vi "Write Housekeeping TS.vi"(8 "error in (no error)":errorcluster, 10 "Housekeeping":i64, 11 "CIFCorePlugin in":refnum<class "CIFCorePlugin.lvclass">) -> (0 "error out":errorcluster, 3 "CIFCorePlugin out":refnum<class "CIFCorePlugin.lvclass">)   [LabVIEW 2021, in "CIFCorePlugin.lvclass"]
doc: "Update the timestamp. Time is U64, absolute time in nS in the appropriate clockID configured for the plugin. If a 0 is wired it will automatically get the current time."
uses:
  CIFCorePlugin.lvclass
  CIFCorePlugin.lvclass/CIFCorePlugin.ctl
  CIFUtilities/CIFClocks/Time Conversion/LabVIEW Time to UTC Time.vi
  Common/Utilities/Add Error.vi
  Common/Utilities/Append Error Location.vi
  <vilib>/CIF Foundation/CIF Utilities/Time/Time_CIF_U.lvlib
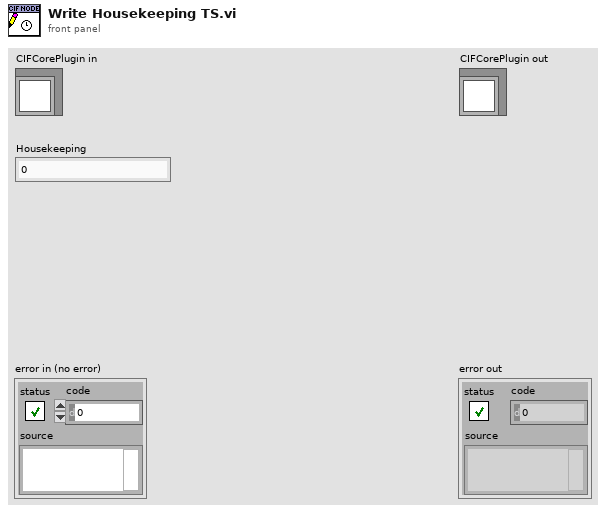
[diagram p1: front panel]
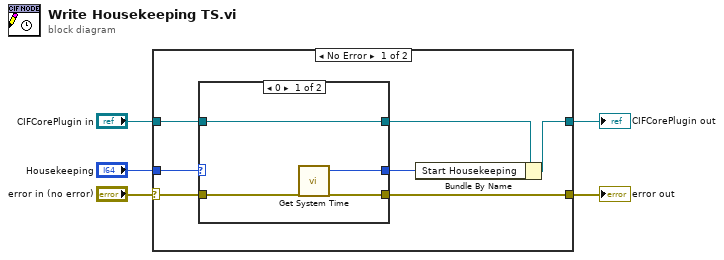
[diagram p0: block diagram]
diagram:
  n1 = case shown="No Error" "error in (no error)" {
    selector: "error in (no error)" -> [w10 w19]
    tunnel: [w6 w19] -> w4
    tunnel: [w12 w20] -> w2
    tunnel: "CIFCorePlugin in" -> [w9 w20]
    tunnel: "Housekeeping" -> [w11 _]
    frame No Error {
      n2 = case shown="0" w11 {
        selector: w11 -> [_ w17]
        tunnel: w10 -> [w13 w16]
        tunnel: w9 -> [w15 w18]
        tunnel: [w15 w18] -> w8
        tunnel: [w14 w17] -> w7
        tunnel: [w13 w16] -> w6
        frame 0 {
          n3 = call <vilib>:"Get System Time.vi"() -> ("Time (ns)"=w14:i64)  [unwired: 5 in]
        }
        frame 1, Default {
        }
      }
      n4 = Bundle By Name(cluster=w8, "Start Housekeeping"=w7) -> (w12:refnum<class "CIFCorePlugin.lvclass">)
    }
    frame Error {
    }
  }
  "error out" <- w4
  "CIFCorePlugin out" <- w2
